vi "SetGainTbl(SubVI).vi"(8 "error in (no error)":errorcluster, 9 "Gain0":dbl caption="Усиление, дБ" min=0.0 max=80.0 step=1.0 format="%.1g", 10 "Tick":i32=1 caption="№ такта" min=1 max=32 step=1, 11 "Gain1":dbl caption="Усиление, дБ" min=0.0 max=80.0 step=1.0 format="%.1g") -> (0 "error out":errorcluster)   [LabVIEW 2017]
uses:
  Global_SNK3_HF.vi
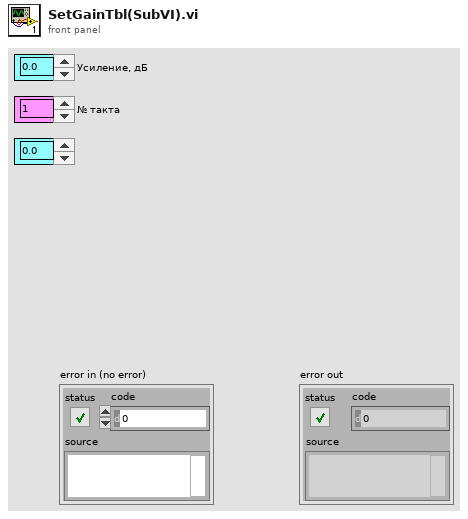
[diagram p1: front panel]
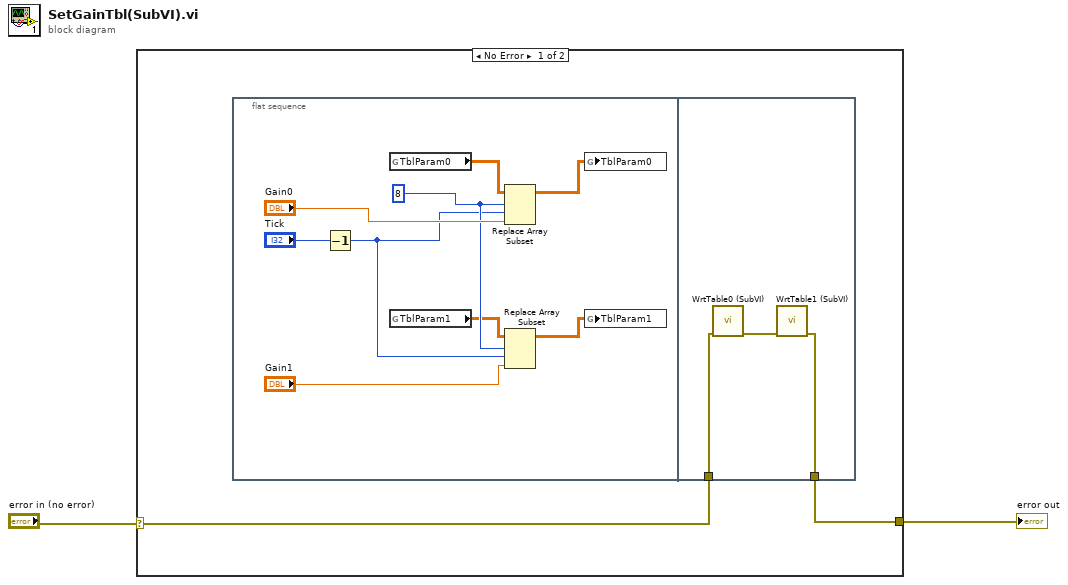
[diagram p0: block diagram]
diagram:
  n1 = case shown="No Error" "error in (no error)" {
    selector: "error in (no error)" -> [w4 w17]
    tunnel: [w3 w17] -> w1
    frame No Error {
      n2 = flat-sequence {
        tunnel: w4 -> [w15]
        tunnel: [w14] -> w3
        frame #0 {
          w10 = 8 ("disabled index (row)")
          n3 = Decrement(x="Tick") -> (x-1=w9:i32)
          n4 = global read "Global_SNK3_HF.vi" "TblParam0"() -> (w6:sgl[][])
          n5 = global read "Global_SNK3_HF.vi" "TblParam1"() -> (w5:sgl[][])
          n6 = Replace Array Subset(array=w6, new element="Gain0", index (row)=w10, index (col)=w9) -> (w7:sgl[][])
          n7 = Replace Array Subset(array=w5, new element="Gain1", index (row)=w10, index (col)=w9) -> (w8:sgl[][])
          n8 = global write "Global_SNK3_HF.vi" "TblParam0"(w7) -> ()
          n9 = global write "Global_SNK3_HF.vi" "TblParam1"(w8) -> ()
        }
        frame #1 {
          n10 = call "WrtTable0 (SubVI).vi"("error in"=w15) -> ("error out"=w16:errorcluster)  [unwired: 10 in]
          n11 = call "WrtTable1 (SubVI).vi"("error in"=w16) -> ("error out"=w14:errorcluster)  [unwired: 10 in]
        }
      }
    }
    frame Error {
    }
  }
  "error out" <- w1
